vi "Folder to 4 digit file.vi"(2 "path 2":path=path "D:/TEST RESULT DATA/2011/PUSHPENDER/November/04/Folder to 4 digit file.vi") -> (0 "decimal integer string":string)   [LabVIEW 2015]
panel:
  out "substring":string
  out "element":string
  out "filenames":string[](array[string])
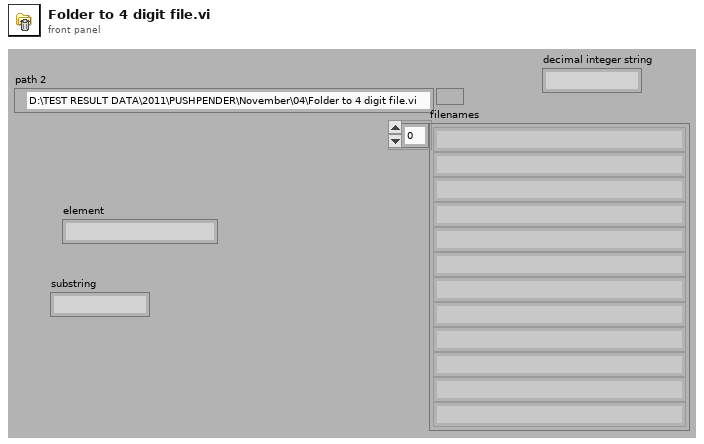
[diagram p1: front panel]
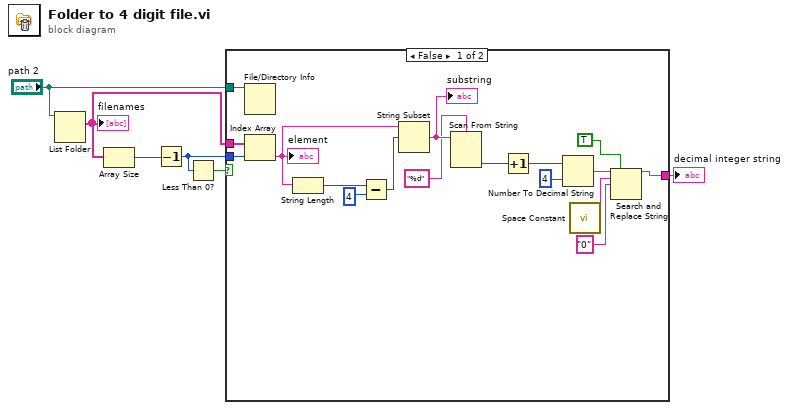
[diagram p0: block diagram]
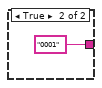
[diagram p2: hidden frame]
diagram:
  n1 = List Folder(path="path 2") -> (filenames=w6:string[])  [unwired: 3 in, 3 out]
  "filenames" <- w6
  n2 = Array Size(array=w6) -> (size(s)=w5:i32)
  n3 = Decrement(x=w5) -> (x-1=w2:i32)
  n4 = Less Than 0?(x=w2) -> (x < 0?=w3:bool)
  n5 = case shown="False" w3 {
    tunnel: w6 -> [w23 _]
    tunnel: w2 -> [w22 _]
    tunnel: [w12 "0001"] -> w4
    tunnel: "path 2" -> [w7 _]
    frame False {
      n6 = File/Directory Info(path=w7) -> ()  [unwired: 1 in, 7 out]
      n7 = Index Array(array=w23, index=w22) -> (element=w21:string)
      "element" <- w21
      n8 = String Length(string=w21) -> (length=w20:i32)
      n9 = Subtract(x=w20, y=4) -> (x-y=w18:i32)
      n10 = String Subset(string=w21, offset (0)=w18) -> (substring=w17:string)  [unwired: 1 in]
      "substring" <- w17
      n11 = Scan From String(format string="%d", input string=w17) -> (output 1=w16:i32)  [unwired: 3 in, 3 out]
      n12 = Increment(x=w16) -> (x+1=w14:i32)
      n13 = Number To Decimal String(number=w14, width (-)=i16 4) -> (decimal integer string=w11:string)
      n14 = call <vilib>:"Space Constant.vi"() -> ("String"=w10:string)
      n15 = Search and Replace String(replace all?=TRUE ("replace all? (F)"), input string=w11, search string=w10, replace string="0" ("replace string (\"\")")) -> (result string=w12:string)  [unwired: 4 in, 3 out]
    }
    frame True {
    }
  }
  "decimal integer string" <- w4
